vi "CSM - Wait and Post Message.vi"(0 "State":string="API State", 1 "Current Module(\"\" to generate a ID)":string, 5 "Arguments (\"\")":string, 7 "Target Module":string="Target", 9 "Wait(5000ms)":i32=5000, 11 "Error In (no error)":errorcluster) -> (15 "error out":errorcluster)   [LabVIEW 2020, in "Communicable State Machine.lvlib"]
doc: "Post a message to CSM specified.\n\n<b>Inputs:</b>\n - <b>Target Module</b>:Target CSM Module name.\n - <b>State</b>: Message to post.\n - <b>Arguments (\"\")</b>: Argument of the message.\n - <b>Error In (no error)</b>: Error cluster\n\n<b>Outputs:</b>\n - <b>error out</b>: Error cluster"
uses:
  Communicable State Machine.lvlib
  Priority Queue.lvclass/Priority Queue.ctl
  uuid.vi
  CSMP-Async Call.vi
  Build Error Cluster.vi
  Trim Both Whitespace.vi
  CSM - Check If Module Exists.vi
  _CSMObj-Message Check.vi
  _CSMObj-Enqueue Cross-Module Message.vi
  _CSMOFGV Get.vi
  _Obtain CSM Data Queue.vi
  Release Priority Queue.vi
  Enqueue Element.vi
  Obtain Priority Queue.vi
  CSM No Target Error.vi
  _CSMOFGV.vi
  CSM Not Allowed Message.vi
  CSM Target Error.vi
  CSM Unhandled State Error.vi
  CSM Target Timeout Error.vi
  Priority Queue.lvclass
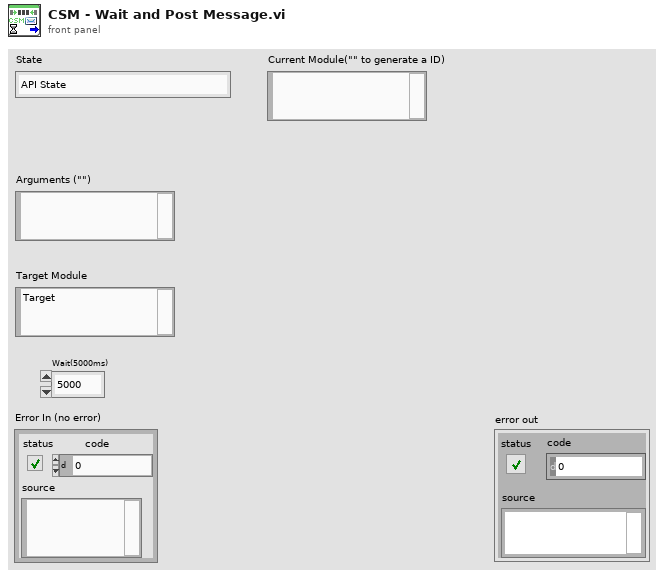
[diagram p1: front panel]
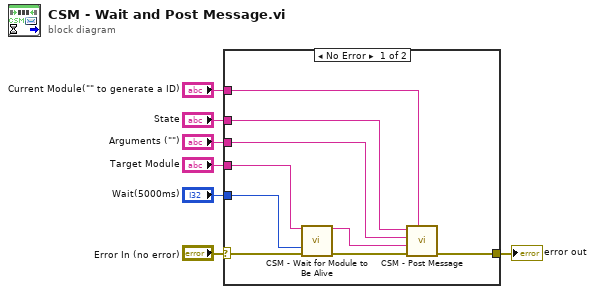
[diagram p0: block diagram]
diagram:
  n1 = case shown="No Error" "Error In (no error)" {
    selector: "Error In (no error)" -> [w10 w17]
    tunnel: "State" -> [w15 _]
    tunnel: [w13 w17] -> w5
    tunnel: "Arguments (\"\")" -> [w14 _]
    tunnel: "Target Module" -> [w11 _]
    tunnel: "Current Module(\"\" to generate a ID)" -> [w16 _]
    tunnel: "Wait(5000ms)" -> [w12 _]
    frame No Error {
      n2 = call "CSM - Wait for Module to Be Alive.vi"("Target Module"=w11, "Wait(5000ms)"=w12, "error in (no error)"=w10) -> ("Target Module (dup)"=w8:string, "error out"=w9:errorcluster)  [unwired: 10 in, 1 out]
      n3 = call "CSM - Post Message.vi"("Current Module(\"\" to generate a ID)"=w16, "Error In (no error)"=w9, "Target Module"=w8, "Arguments (\"\")"=w14, "State"=w15) -> ("error out"=w13:errorcluster)  [unwired: 6 in]
    }
    frame Error {
    }
  }
  "error out" <- w5
